vi "Check Variable Name Valid.vi"(1 "String":string) -> (0 "Boolean":bool)   [LabVIEW 2015, in "Project.lvclass"]
uses:
  Project.lvclass
  <vilib>/regexp/Match Regular Expression.xnode
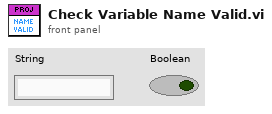
[diagram p1: front panel]
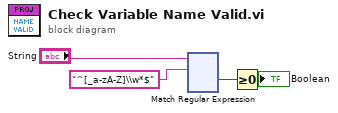
[diagram p0: block diagram]
diagram:
  n1 = xnode "Match Regular Expression"("input string"="String", "regular expression"="^[_a-zA-Z]\\w*$") -> ("offset past match"=w2:i32)  [unwired: 4 in, 4 out]
  n2 = Greater Or Equal To 0?(x=w2) -> (x >= 0?=→"Boolean":bool)
